vi "Experiment_manager.vi"(0 "Enum":T1(ring), 5 "N":dbl, 7 "Stoplive":bool, 9 "Acq Trigger":bool, 11 "end":bool) -> (4 "Even":dbl[][](array[numeric]), 6 "Odd":dbl[][](array[numeric]))   [LabVIEW 2026]
panel:
  out "Intensity Graph 2":dbl[][](graph)
  out "Intensity Graph":dbl[][](graph)
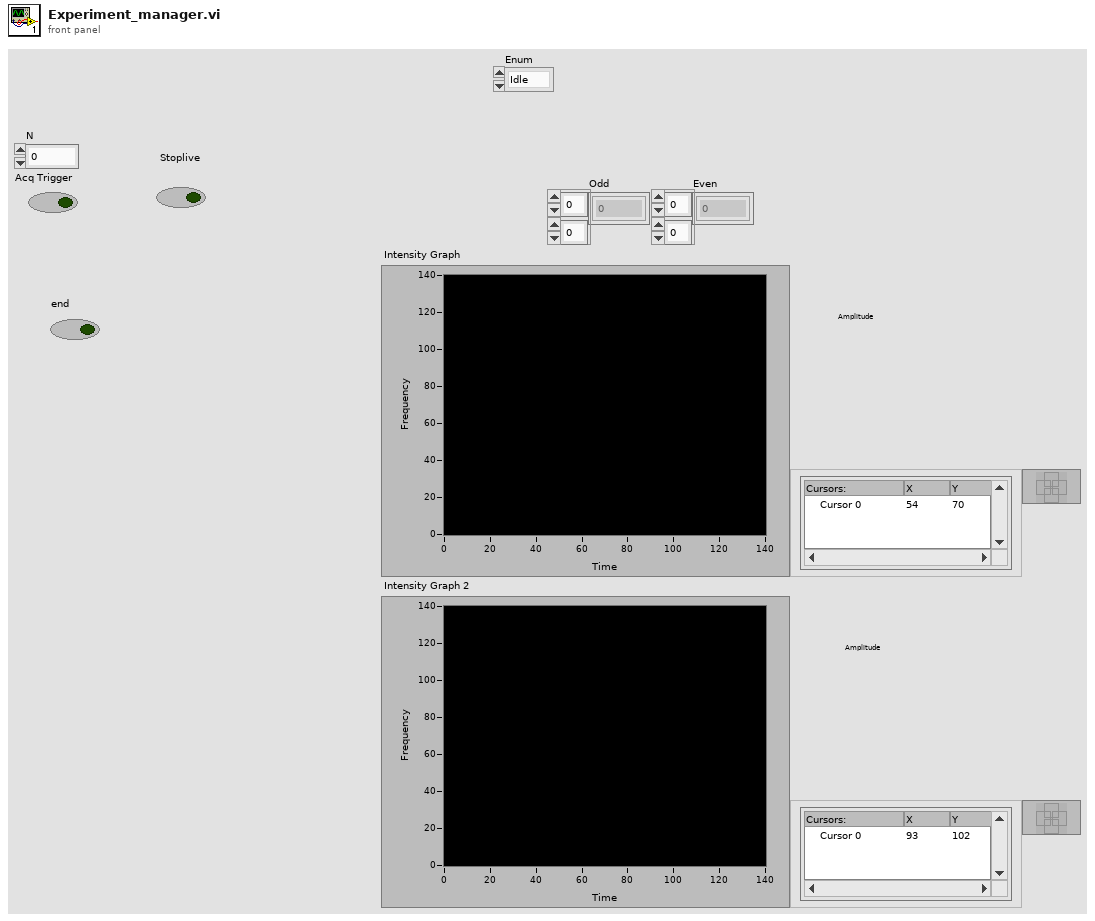
[diagram p1: front panel]
types:
  T1 = enum16{"Idle", "Init", "Getframe", "Close", "Measure"}
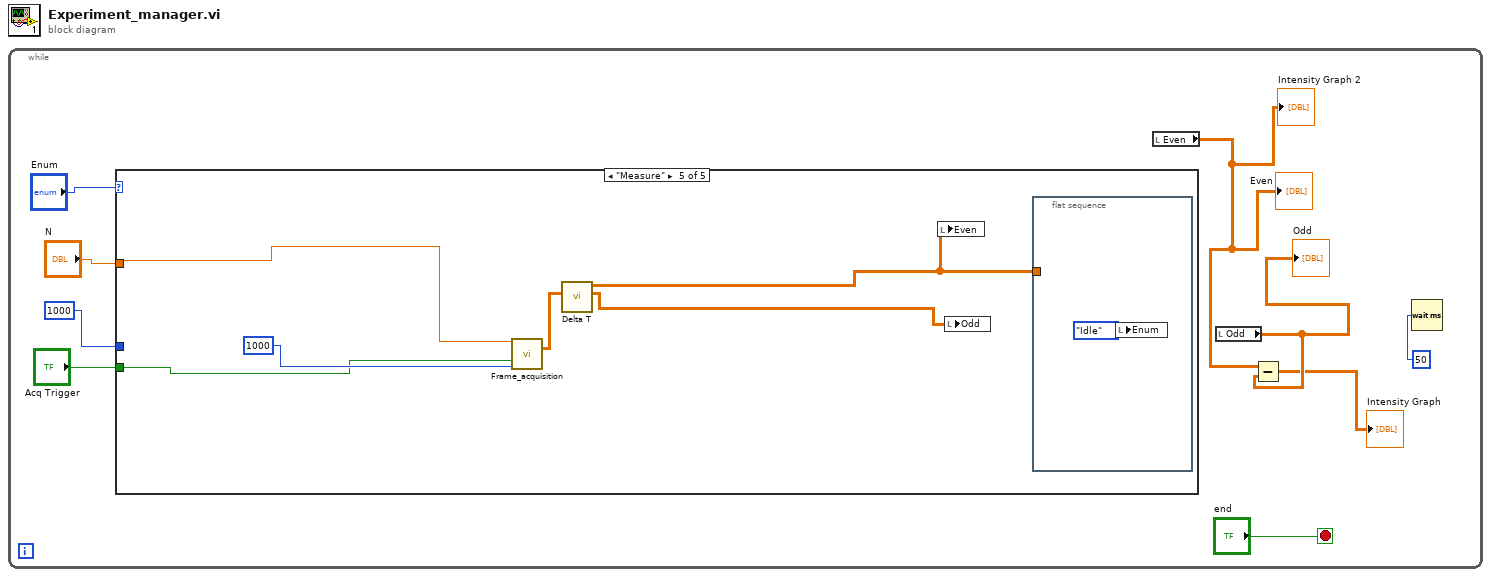
[diagram p0: block diagram]
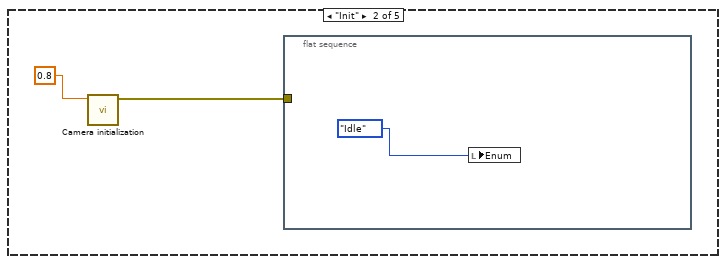
[diagram p3: hidden frame]
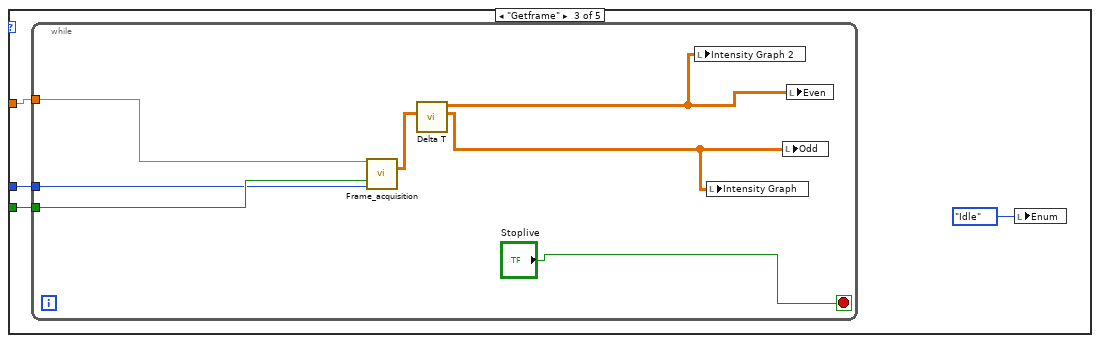
[diagram p4: hidden frame]
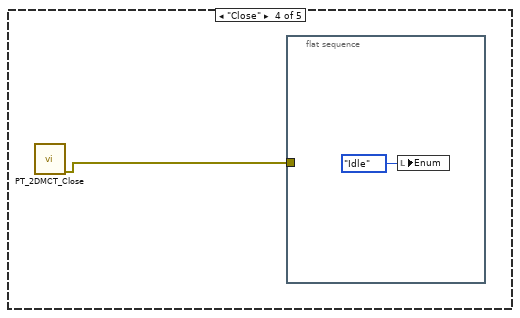
[diagram p5: hidden frame]
diagram:
  n1 = while {
    stop <- "end" stop-if-true
    n2 = case shown="\"Measure\"" "Enum" {
      tunnel: "Acq Trigger" -> [_ _ w15 _ w28]
      tunnel: "N" -> [_ _ w16 _ w29]
      tunnel: 1000 -> [_ _ w13 _ _]
      frame "Idle", Default {
      }
      frame "Init" {
        n3 = call "Camera initialization.vi"("IntegrationTime (us)"=0.8) -> ("error out"=w10:errorcluster)  [unwired: 8 in, 2 out]
        n4 = flat-sequence {
          tunnel: w10 -> [_]
          frame #0 {
            n5 = local write "Enum"(enum16{"Idle", "Init", "Getframe", "Close"}."Idle" ("Enum")) -> ()
          }
        }
      }
      frame "Getframe" {
        n6 = while {
          tunnel: w16 -> [w21]
          tunnel: w15 -> [w20]
          tunnel: w13 -> [w19]
          stop <- "Stoplive" stop-if-true
          n7 = call "Frame_acquisition.vi"("Frames"=w21, "Acq Trigger?"=w20, "Timeout"=w19) -> ("FrameData"=w23:dbl[][][])  [unwired: 11 in, 1 out]
          n8 = call "Delta T.vi"("FrameData"=w23) -> ("Odd"=w17:dbl[][], "Even"=w18:dbl[][])  [unwired: 7 in, 2 out]
          n9 = local write "Intensity Graph 2"(w18) -> ()
          n10 = local write "Intensity Graph"(w17) -> ()
          n11 = local write "Odd"(w17) -> ()
          n12 = local write "Even"(w18) -> ()
        }
        n13 = local write "Enum"(T1."Idle" ("Enum")) -> ()
      }
      frame "Close" {
        n14 = call "PT_2DMCT_Close.vi"() -> ("error out"=w24:errorcluster)  [unwired: 11 in]
        n15 = flat-sequence {
          tunnel: w24 -> [_]
          frame #0 {
            n16 = local write "Enum"(T1."Idle" ("Enum")) -> ()
          }
        }
      }
      frame "Measure" {
        n17 = call "Frame_acquisition.vi"("Frames"=w29, "Acq Trigger?"=w28, "Timeout"=1000) -> ("FrameData"=w31:dbl[][][])  [unwired: 11 in, 1 out]
        n18 = call "Delta T.vi"("FrameData"=w31) -> ("Odd"=w27:dbl[][], "Even"=w26:dbl[][])  [unwired: 7 in, 2 out]
        n19 = local write "Even"(w26) -> ()
        n20 = local write "Odd"(w27) -> ()
        n21 = flat-sequence {
          tunnel: w26 -> [_]
          frame #0 {
            n22 = local write "Enum"(T1."Idle" ("Enum")) -> ()
          }
        }
      }
    }
    n23 = local read "Even"() -> (w3:dbl[][])
    "Even" <- w3
    "Intensity Graph 2" <- w3
    n24 = local read "Odd"() -> (w2:dbl[][])
    "Odd" <- w2
    n25 = Subtract(x=w3, y=w2) -> (x-y=→"Intensity Graph":dbl[][])
    n26 = Wait (ms)(milliseconds to wait=u32 50) -> ()  [unwired: 1 out]
  }
